vi "SP Convert 4.0 - 4.1 to 4.2.vi"(0 "S Parameter 4.0 - 4.1 Test Parameters":T3={"Tag"="", "Stimulus"={"Use Instrument Settings"=FALSE, "Sweep Type"=enum."Linear", "Sweep"=[{"Fstart, MHz"=500.0, "Fstop, MHz"=1500.0, "Points"=201}], "Blank Frequencies"=FALSE, "Power, dBm"=999.0, "IFBW, Hz"=-1.0, "Sweep Time, s"=-1.0}, "Measurements"=[{"Channel"=0, "Parameters"=[]}], "Datasheets"={"Datasheets to Generate"=[], "Print Datasheets"=FALSE}, "Quick Mode"=FALSE, "Display"={"Retain Settings"=FALSE, "Lock Control"=FALSE, "Plot Orientation"=enum."Single", "CH Controls"=[{"Trace Orientation"=enum."Overlay", "Frequency"={"Start"=500.0, "Stop"=1500.0, "Units"="MHz"}, "CH1Control"={"ChOn"=TRUE, "Measure"=0, "Format"=0, "Autoscale"=TRUE, "Reference"=0.0, "\nRefUnit"="dB/Div", "Position"=5.0, "Scale"=10.0, "ScaleUnit"="dB/Div", "LimitOn"=TRUE, "LimitFill"=FALSE, "Display Data"=0, "Show Markers"=FALSE, "SXX"=""}, "CH2Control"={"ChOn"=TRUE, "Measure"=0, "Format"=0, "Autoscale"=TRUE, "Reference"=0.0, "\nRefUnit"="dB/Div", "Position"=5.0, "Scale"=10.0, "ScaleUnit"="dB/Div", "LimitOn"=TRUE, "LimitFill"=FALSE, "Display Data"=0, "Show Markers"=FALSE, "SXX"=""}, "Markers"=[]}, {"Trace Orientation"=enum."Overlay", "Frequency"={"Start"=500.0, "Stop"=1500.0, "Units"="MHz"}, "CH1Control"={"ChOn"=TRUE, "Measure"=0, "Format"=0, "Autoscale"=TRUE, "Reference"=0.0, "\nRefUnit"="dB/Div", "Position"=5.0, "Scale"=10.0, "ScaleUnit"="dB/Div", "LimitOn"=TRUE, "LimitFill"=FALSE, "Display Data"=0, "Show Markers"=FALSE, "SXX"=""}, "CH2Control"={"ChOn"=TRUE, "Measure"=0, "Format"=0, "Autoscale"=TRUE, "Reference"=0.0, "\nRefUnit"="dB/Div", "Position"=5.0, "Scale"=10.0, "ScaleUnit"="dB/Div", "LimitOn"=TRUE, "LimitFill"=FALSE, "Display Data"=0, "Show Markers"=FALSE, "SXX"=""}, "Markers"=[]}, {"Trace Orientation"=enum."Overlay", "Frequency"={"Start"=500.0, "Stop"=1500.0, "Units"="MHz"}, "CH1Control"={"ChOn"=TRUE, "Measure"=0, "Format"=0, "Autoscale"=TRUE, "Reference"=0.0, "\nRefUnit"="dB/Div", "Position"=5.0, "Scale"=10.0, "ScaleUnit"="dB/Div", "LimitOn"=TRUE, "LimitFill"=FALSE, "Display Data"=0, "Show Markers"=FALSE, "SXX"=""}, "CH2Control"={"ChOn"=TRUE, "Measure"=0, "Format"=0, "Autoscale"=TRUE, "Reference"=0.0, "\nRefUnit"="dB/Div", "Position"=5.0, "Scale"=10.0, "ScaleUnit"="dB/Div", "LimitOn"=TRUE, "LimitFill"=FALSE, "Display Data"=0, "Show Markers"=FALSE, "SXX"=""}, "Markers"=[]}, {"Trace Orientation"=enum."Overlay", "Frequency"={"Start"=500.0, "Stop"=1500.0, "Units"="MHz"}, "CH1Control"={"ChOn"=TRUE, "Measure"=0, "Format"=0, "Autoscale"=TRUE, "Reference"=0.0, "\nRefUnit"="dB/Div", "Position"=5.0, "Scale"=10.0, "ScaleUnit"="dB/Div", "LimitOn"=TRUE, "LimitFill"=FALSE, "Display Data"=0, "Show Markers"=FALSE, "SXX"=""}, "CH2Control"={"ChOn"=TRUE, "Measure"=0, "Format"=0, "Autoscale"=TRUE, "Reference"=0.0, "\nRefUnit"="dB/Div", "Position"=5.0, "Scale"=10.0, "ScaleUnit"="dB/Div", "LimitOn"=TRUE, "LimitFill"=FALSE, "Display Data"=0, "Show Markers"=FALSE, "SXX"=""}, "Markers"=[]}], "Formatted Data"=FALSE}, "Auto Select"=TRUE, "Calibration"={"State"=FALSE, "String"=""}} {"Stimulus"."Sweep Time, s" format="%.3g"; "Display"."CH Controls"."Frequency"."Stop" format="%.3g"; "Display"."CH Controls"."Frequency"."Start" format="%.3g"; "Display"."CH Controls"."CH2Control"."Reference" format="%#.2g"; "Display"."CH Controls"."CH2Control"."Display Data" items=["Data", "Memory", "Data/Memory"]; "Display"."CH Controls"."CH2Control"."Format" items=["Log Mag", "Phase", "Delay", "Smith", "Polar", "Lin Mag", "SWR", "Loss", "Real", "Imaginary"]; "Display"."CH Controls"."CH2Control"."Scale" min=0.001 step=1.0 format="%#.2g"; "Display"."CH Controls"."CH2Control"."Position" min=0.0 max=10.0; "Display"."CH Controls"."CH1Control"."Reference" format="%#.2g"; "Display"."CH Controls"."CH1Control"."Display Data" items=["Data", "Memory", "Data/Memory"]; "Display"."CH Controls"."CH1Control"."Format" items=["Log Mag", "Phase", "Delay", "Smith", "Polar", "Lin Mag", "SWR", "Loss", "Real", "Imaginary"]; "Display"."CH Controls"."CH1Control"."Scale" min=0.001 step=1.0 format="%#.2g"; "Display"."CH Controls"."CH1Control"."Position" min=0.0 max=10.0; "Measurements"."Parameters"."Limits"."Run" min=1 step=1; "Measurements"."Channel" min=0 max=32 step=1}) -> (1 "QuickMode":i8, 2 "S Parameter 4.2 Test Parameters":T2={"Stimulus"={"Use Instrument Settings"=FALSE, "Blank Frequencies"=FALSE, "Sweep Type"=enum."Linear", "Sweep"={"Fstart"=0.0, "Fstop"=0.0, "Units"=enum."Hz", "Points"=2}, "Power (dBm)"=999.0, "IFBW (Hz)"=-1.0, "Sweep Time (s)"=-1.0}, "Measurement"={"Auto Select"=TRUE, "Data Source"=enum."VNA", "Ports"=2, "Calibration"={"State"=FALSE, "String"=""}, "Parameters"=[]}, "De-Embed"={"De-Embed"=FALSE, "Adapters"=[]}, "Display"={"Lock Control"=FALSE, "Retain Settings"=TRUE, "Formatted Data"=FALSE, "Plot Orientation"=enum."Single", "Plot Controls"=[{"Trace Orientation"=enum."Overlay", "Frequency"={"Change Frequency"=FALSE, "Start"=500.0, "Stop"=1500.0, "Units"=enum."MHz"}, "Markers (MHz)"=[], "Traces"=[{"Trace On"=TRUE, "Measure"=0, "Format"=0, "Autoscale"=TRUE, "Reference"=0.0, "\nRefUnit"="dB/Div", "Position"=5.0, "Scale"=10.0, "ScaleUnit"="dB/Div", "LimitOn"=TRUE, "LimitFill"=FALSE, "Display Data"=0, "Show Markers"=FALSE, "SXX"=""}, {"Trace On"=TRUE, "Measure"=0, "Format"=0, "Autoscale"=TRUE, "Reference"=0.0, "\nRefUnit"="dB/Div", "Position"=5.0, "Scale"=10.0, "ScaleUnit"="dB/Div", "LimitOn"=TRUE, "LimitFill"=FALSE, "Display Data"=0, "Show Markers"=FALSE, "SXX"=""}]}, {"Trace Orientation"=enum."Overlay", "Frequency"={"Change Frequency"=FALSE, "Start"=500.0, "Stop"=1500.0, "Units"=enum."MHz"}, "Markers (MHz)"=[], "Traces"=[{"Trace On"=TRUE, "Measure"=0, "Format"=0, "Autoscale"=TRUE, "Reference"=0.0, "\nRefUnit"="dB/Div", "Position"=5.0, "Scale"=10.0, "ScaleUnit"="dB/Div", "LimitOn"=TRUE, "LimitFill"=FALSE, "Display Data"=0, "Show Markers"=FALSE, "SXX"=""}, {"Trace On"=TRUE, "Measure"=0, "Format"=0, "Autoscale"=TRUE, "Reference"=0.0, "\nRefUnit"="dB/Div", "Position"=5.0, "Scale"=10.0, "ScaleUnit"="dB/Div", "LimitOn"=TRUE, "LimitFill"=FALSE, "Display Data"=0, "Show Markers"=FALSE, "SXX"=""}]}, {"Trace Orientation"=enum."Overlay", "Frequency"={"Change Frequency"=FALSE, "Start"=500.0, "Stop"=1500.0, "Units"=enum."MHz"}, "Markers (MHz)"=[], "Traces"=[{"Trace On"=TRUE, "Measure"=0, "Format"=0, "Autoscale"=TRUE, "Reference"=0.0, "\nRefUnit"="dB/Div", "Position"=5.0, "Scale"=10.0, "ScaleUnit"="dB/Div", "LimitOn"=TRUE, "LimitFill"=FALSE, "Display Data"=0, "Show Markers"=FALSE, "SXX"=""}, {"Trace On"=TRUE, "Measure"=0, "Format"=0, "Autoscale"=TRUE, "Reference"=0.0, "\nRefUnit"="dB/Div", "Position"=5.0, "Scale"=10.0, "ScaleUnit"="dB/Div", "LimitOn"=TRUE, "LimitFill"=FALSE, "Display Data"=0, "Show Markers"=FALSE, "SXX"=""}]}, {"Trace Orientation"=enum."Overlay", "Frequency"={"Change Frequency"=FALSE, "Start"=500.0, "Stop"=1500.0, "Units"=enum."MHz"}, "Markers (MHz)"=[], "Traces"=[{"Trace On"=TRUE, "Measure"=0, "Format"=0, "Autoscale"=TRUE, "Reference"=0.0, "\nRefUnit"="dB/Div", "Position"=5.0, "Scale"=10.0, "ScaleUnit"="dB/Div", "LimitOn"=TRUE, "LimitFill"=FALSE, "Display Data"=0, "Show Markers"=FALSE, "SXX"=""}, {"Trace On"=TRUE, "Measure"=0, "Format"=0, "Autoscale"=TRUE, "Reference"=0.0, "\nRefUnit"="dB/Div", "Position"=5.0, "Scale"=10.0, "ScaleUnit"="dB/Div", "LimitOn"=TRUE, "LimitFill"=FALSE, "Display Data"=0, "Show Markers"=FALSE, "SXX"=""}]}]}, "Limits"=[], "Datasheets"=[]} {"Measurement"."Parameters"."Channel" min=0 max=32 step=1; "Stimulus"."Sweep Time (s)" format="%.3g"; "Display"."Plot Controls"."Traces"."Reference" format="%#.2g"; "Display"."Plot Controls"."Traces"."Display Data" items=["Data", "Memory", "Data/Memory"]; "Display"."Plot Controls"."Traces"."Format" items=["Log Mag", "Phase", "Delay", "Smith", "Polar", "Lin Mag", "SWR", "Loss", "Real", "Imaginary"]; "Display"."Plot Controls"."Traces"."Scale" min=0.001 step=1.0 format="%#.2g"; "Display"."Plot Controls"."Traces"."Position" min=0.0 max=10.0; "Display"."Plot Controls"."Frequency"."Stop" format="%.3g"; "Display"."Plot Controls"."Frequency"."Start" format="%.3g"})   [LabVIEW 2011]
uses:
  TypeDefs/SP Test Parameters v3.2 and 4.0-4.1.ctl
  TypeDefs/SP Test Parameters v4.2.ctl
  TypeDefs/SP Format.ctl
panel:
  in  "Format":T1
  # "Div"
  # "Div"
  # "Div"
  # "="
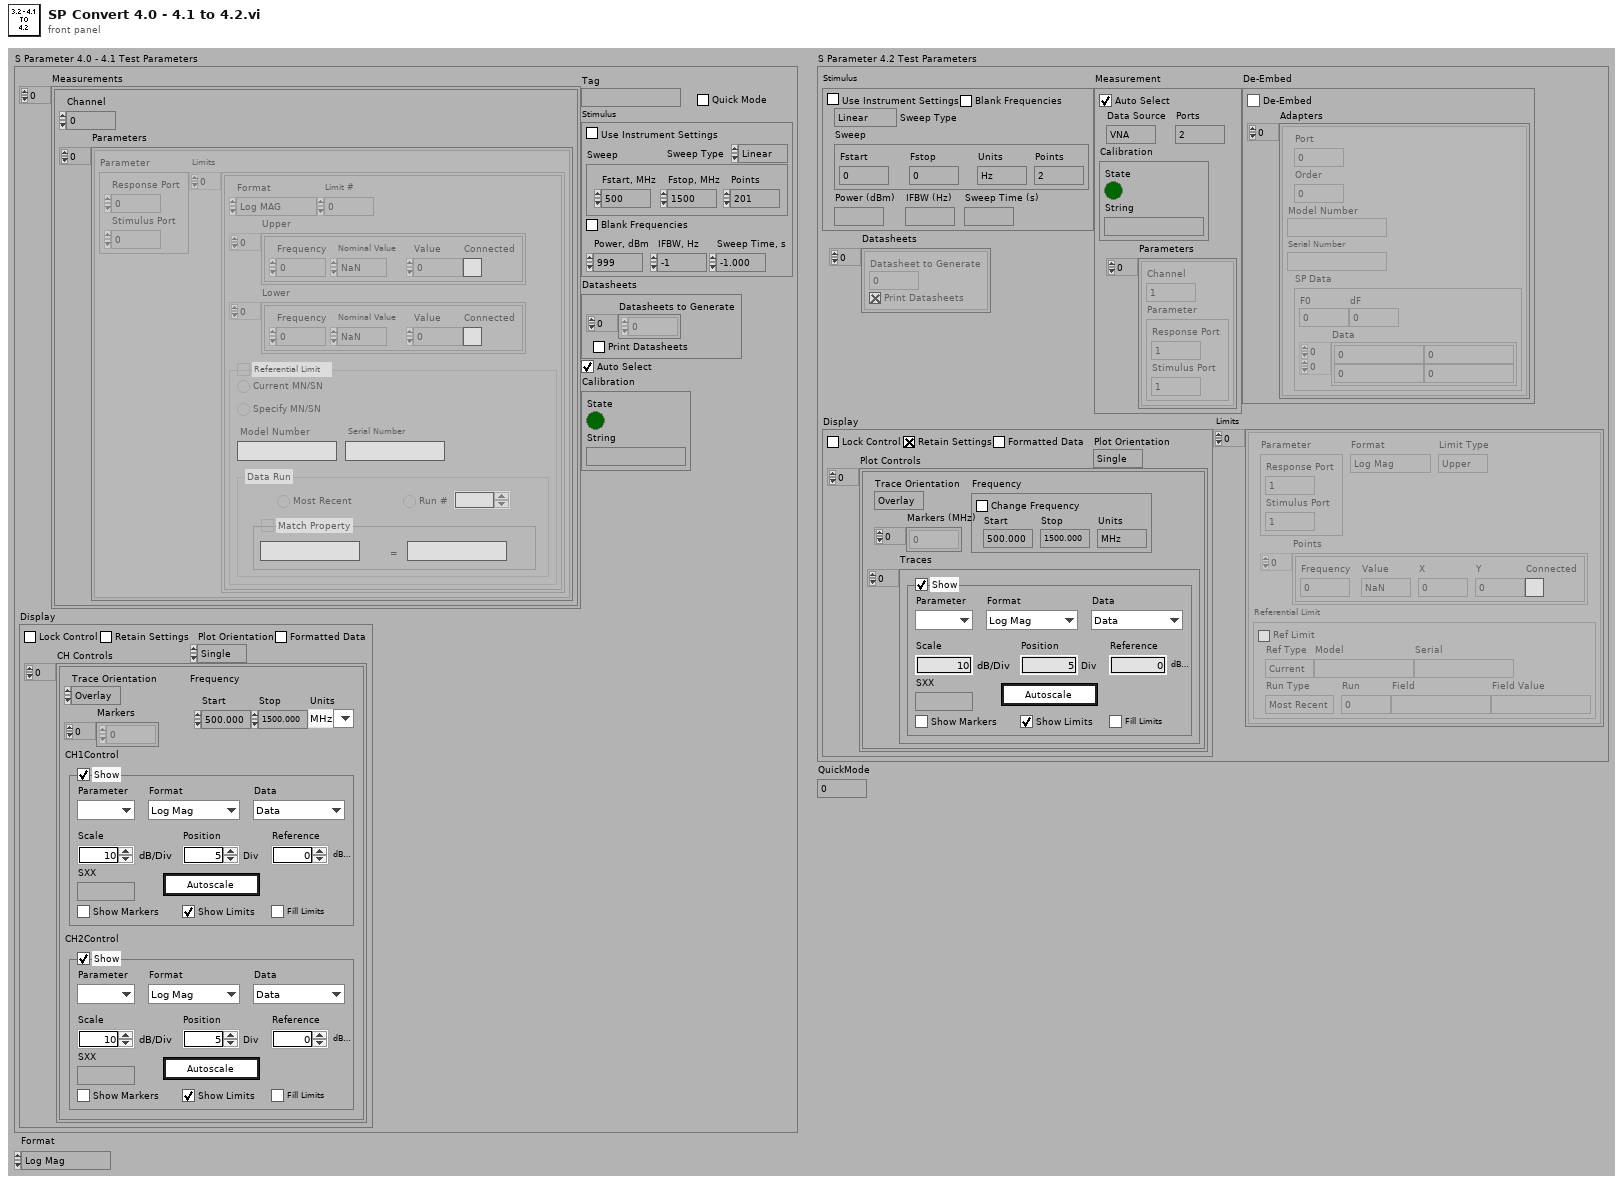
[diagram p1: front panel]
types:
  T1 = typedef "SP Format.ctl" = enum16{"Log Mag", "Lin Mag", "SWR", "Phase", "Expanded Phase", "Delay", "Insertion Loss", "Isolation", "Return Loss"}
  T2 = typedef "SP Test Parameters v4.2.ctl" = cluster{"Stimulus":cluster{"Use Instrument Settings":bool, "Blank Frequencies":bool, "Sweep Type":enum32{"Linear", "Logarithmic", "List", "Power", "CW"}, "Sweep":cluster{"Fstart":dbl, "Fstop":dbl, "Units":enum16{"Hz", "kHz", "MHz", "GHz"}, "Points":i32}, "Power (dBm)":dbl, "IFBW (Hz)":dbl, "Sweep Time (s)":dbl}, "Measurement":cluster{"Auto Select":bool, "Data Source":enum16{"VNA", "Data File"}, "Ports":i8, "Calibration":cluster{"State":bool, "String":string}, "Parameters":cluster{"Channel":i8, "Parameter":cluster{"Stimulus Port":i8, "Response Port":i8}}[]}, "De-Embed":cluster{"De-Embed":bool, "Adapters":cluster{"Port":i8, "Order":i8, "Model Number":string, "Serial Number":string, "SP Data":cluster{"F0":dbl, "dF":dbl, "Data":cdb[][]}}[]}, "Display":cluster{"Lock Control":bool, "Retain Settings":bool, "Formatted Data":bool, "Plot Orientation":enum32{"Single", "Dual", "Quad"}, "Plot Controls":cluster{"Trace Orientation":enum32{"Overlay", "Split"}, "Frequency":cluster{"Change Frequency":bool, "Start":dbl, "Stop":dbl, "Units":enum16{"Hz", "kHz", "MHz", "GHz"}}, "Markers (MHz)":dbl[], "Traces":cluster{"Trace On":bool, "Measure":i32, "Format":i32, "Autoscale":bool, "Reference":dbl, "\nRefUnit":string, "Position":dbl, "Scale":dbl, "ScaleUnit":string, "LimitOn":bool, "LimitFill":bool, "Display Data":u16, "Show Markers":bool, "SXX":string}[]}[]}, "Limits":cluster{"Parameter":cluster{"Stimulus Port":i8, "Response Port":i8}, "Format":enum16{"Log Mag", "Lin Mag", "SWR", "Phase", "Delay", "Insertion Loss", "Isolation", "Return Loss"}, "Limit Type":enum16{"Upper", "Lower", "Delta"}, "Points":cluster{"Frequency":dbl, "Value":dbl, "X":dbl, "Y":dbl, "Connected":bool}[], "Referential Limit":cluster{"Ref Limit":bool, "Ref Type":enum16{"Current", "Specify"}, "Model":string, "Serial":string, "Run Type":enum16{"Most Recent", "Run #", "Match Field"}, "Run":i32, "Field":string, "Field Value":string}}[], "Datasheets":cluster{"Datasheet to Generate":i32, "Print Datasheets":bool}[]}
  T3 = typedef "SP Test Parameters v3.2 and 4.0-4.1.ctl" = cluster{"Tag":string, "Stimulus":cluster{"Use Instrument Settings":bool, "Sweep Type":enum32{"Linear", "Log", "List", "Power", "CW"}, "Sweep":cluster{"Fstart, MHz":dbl, "Fstop, MHz":dbl, "Points":i32}[], "Blank Frequencies":bool, "Power, dBm":dbl, "IFBW, Hz":dbl, "Sweep Time, s":dbl}, "Measurements":cluster{"Channel":i8, "Parameters":cluster{"Parameter":cluster{"Stimulus Port":i8, "Response Port":i8}, "Limits":cluster{"Format":enum16{"Log MAG", "Lin MAG", "VSWR", "Phase", "Delay", "Insertion Loss", "Isolation", "Return Loss"}, "Upper":cluster{"Frequency":dbl, "Nominal Value":dbl, "Value":dbl, "Connected":bool}[], "Lower":cluster{"Frequency":dbl, "Nominal Value":dbl, "Value":dbl, "Connected":bool}[], "Limit #":i32, "Ref Limit":bool, "Ref Type":enum32{"Current", "Specify"}, "Model":string, "Serial":string, "Run Type":enum32{"Most Recent", "Run #"}, "Run":i32, "Match Property":bool, "Property":string, "Property Value":string}[]}[]}[], "Datasheets":cluster{"Datasheets to Generate":i32[], "Print Datasheets":bool}, "Quick Mode":bool, "Display":cluster{"Retain Settings":bool, "Lock Control":bool, "Plot Orientation":enum32{"Single", "Dual", "Quad"}, "CH Controls":cluster{"Trace Orientation":enum32{"Overlay", "Split"}, "Frequency":cluster{"Start":dbl, "Stop":dbl, "Units":string}, "CH1Control":cluster{"ChOn":bool, "Measure":i32, "Format":i32, "Autoscale":bool, "Reference":dbl, "\nRefUnit":string, "Position":dbl, "Scale":dbl, "ScaleUnit":string, "LimitOn":bool, "LimitFill":bool, "Display Data":u16, "Show Markers":bool, "SXX":string}, "CH2Control":cluster{"ChOn":bool, "Measure":i32, "Format":i32, "Autoscale":bool, "Reference":dbl, "\nRefUnit":string, "Position":dbl, "Scale":dbl, "ScaleUnit":string, "LimitOn":bool, "LimitFill":bool, "Display Data":u16, "Show Markers":bool, "SXX":string}, "Markers":dbl[]}[], "Formatted Data":bool}, "Auto Select":bool, "Calibration":cluster{"State":bool, "String":string}}
  T4 = enum32{"Linear", "Logarithmic", "List", "Power", "CW"}
  T5 = cluster{"Datasheet to Generate":i32, "Print Datasheets":bool}[]
  T6 = cluster{"Trace Orientation":enum32{"Overlay", "Split"}, "Frequency":cluster{"Change Frequency":bool, "Start":dbl, "Stop":dbl, "Units":enum16{"Hz", "kHz", "MHz", "GHz"}}, "Markers (MHz)":dbl[], "Traces":cluster{"Trace On":bool, "Measure":i32, "Format":i32, "Autoscale":bool, "Reference":dbl, "\nRefUnit":string, "Position":dbl, "Scale":dbl, "ScaleUnit":string, "LimitOn":bool, "LimitFill":bool, "Display Data":u16, "Show Markers":bool, "SXX":string}[]}[]
  T7 = cluster{"Channel":i8, "Parameter":cluster{"Stimulus Port":i8, "Response Port":i8}}[]
  T8 = cluster{"Parameter":cluster{"Stimulus Port":i8, "Response Port":i8}, "Format":enum16{"Log Mag", "Lin Mag", "SWR", "Phase", "Delay", "Insertion Loss", "Isolation", "Return Loss"}, "Limit Type":enum16{"Upper", "Lower", "Delta"}, "Points":cluster{"Frequency":dbl, "Value":dbl, "X":dbl, "Y":dbl, "Connected":bool}[], "Referential Limit":cluster{"Ref Limit":bool, "Ref Type":enum16{"Current", "Specify"}, "Model":string, "Serial":string, "Run Type":enum16{"Most Recent", "Run #", "Match Field"}, "Run":i32, "Field":string, "Field Value":string}}[]
  T9 = cluster{"Parameter":cluster{"Stimulus Port":i8, "Response Port":i8}, "Format":enum16{"Log Mag", "Lin Mag", "SWR", "Phase", "Delay", "Insertion Loss", "Isolation", "Return Loss"}, "Limit Type":enum16{"Upper", "Lower", "Delta"}, "Points":cluster{"Frequency":dbl, "Value":dbl, "X":dbl, "Y":dbl, "Connected":bool}[], "Referential Limit":cluster{"Ref Limit":bool, "Ref Type":enum16{"Current", "Specify"}, "Model":string, "Serial":string, "Run Type":enum16{"Most Recent", "Run #", "Match Field"}, "Run":i32, "Field":string, "Field Value":string}}
  T10 = cluster{"Frequency":dbl, "Value":dbl, "X":dbl, "Y":dbl, "Connected":bool}[]
  T11 = cluster{"Trace Orientation":enum32{"Overlay", "Split"}, "Frequency":cluster{"Change Frequency":bool, "Start":dbl, "Stop":dbl, "Units":enum16{"Hz", "kHz", "MHz", "GHz"}}, "Markers (MHz)":dbl[], "Traces":cluster{"Trace On":bool, "Measure":i32, "Format":i32, "Autoscale":bool, "Reference":dbl, "\nRefUnit":string, "Position":dbl, "Scale":dbl, "ScaleUnit":string, "LimitOn":bool, "LimitFill":bool, "Display Data":u16, "Show Markers":bool, "SXX":string}[]}
  T12 = cluster{"Fstart, MHz":dbl, "Fstop, MHz":dbl, "Points":i32}[]
  T13 = cluster{"Datasheets to Generate":i32[], "Print Datasheets":bool}
  T14 = cluster{"Trace Orientation":enum32{"Overlay", "Split"}, "Frequency":cluster{"Start":dbl, "Stop":dbl, "Units":string}, "CH1Control":cluster{"ChOn":bool, "Measure":i32, "Format":i32, "Autoscale":bool, "Reference":dbl, "\nRefUnit":string, "Position":dbl, "Scale":dbl, "ScaleUnit":string, "LimitOn":bool, "LimitFill":bool, "Display Data":u16, "Show Markers":bool, "SXX":string}, "CH2Control":cluster{"ChOn":bool, "Measure":i32, "Format":i32, "Autoscale":bool, "Reference":dbl, "\nRefUnit":string, "Position":dbl, "Scale":dbl, "ScaleUnit":string, "LimitOn":bool, "LimitFill":bool, "Display Data":u16, "Show Markers":bool, "SXX":string}, "Markers":dbl[]}[]
  T15 = cluster{"Channel":i8, "Parameters":cluster{"Parameter":cluster{"Stimulus Port":i8, "Response Port":i8}, "Limits":cluster{"Format":enum16{"Log MAG", "Lin MAG", "VSWR", "Phase", "Delay", "Insertion Loss", "Isolation", "Return Loss"}, "Upper":cluster{"Frequency":dbl, "Nominal Value":dbl, "Value":dbl, "Connected":bool}[], "Lower":cluster{"Frequency":dbl, "Nominal Value":dbl, "Value":dbl, "Connected":bool}[], "Limit #":i32, "Ref Limit":bool, "Ref Type":enum32{"Current", "Specify"}, "Model":string, "Serial":string, "Run Type":enum32{"Most Recent", "Run #"}, "Run":i32, "Match Property":bool, "Property":string, "Property Value":string}[]}[]}[]
  T16 = cluster{"Trace On":bool, "Measure":i32, "Format":i32, "Autoscale":bool, "Reference":dbl, "\nRefUnit":string, "Position":dbl, "Scale":dbl, "ScaleUnit":string, "LimitOn":bool, "LimitFill":bool, "Display Data":u16, "Show Markers":bool, "SXX":string}[]
  T17 = cluster{"Frequency":dbl, "Value":dbl, "X":dbl, "Y":dbl, "Connected":bool}
  T18 = cluster{"Channel":i8, "Parameter":cluster{"Stimulus Port":i8, "Response Port":i8}}
  T19 = enum16{"Log Mag", "Lin Mag", "SWR", "Phase", "Delay", "Insertion Loss", "Isolation", "Return Loss"}
  T20 = cluster{"Parameter":cluster{"Stimulus Port":i8, "Response Port":i8}, "Limits":cluster{"Format":enum16{"Log MAG", "Lin MAG", "VSWR", "Phase", "Delay", "Insertion Loss", "Isolation", "Return Loss"}, "Upper":cluster{"Frequency":dbl, "Nominal Value":dbl, "Value":dbl, "Connected":bool}[], "Lower":cluster{"Frequency":dbl, "Nominal Value":dbl, "Value":dbl, "Connected":bool}[], "Limit #":i32, "Ref Limit":bool, "Ref Type":enum32{"Current", "Specify"}, "Model":string, "Serial":string, "Run Type":enum32{"Most Recent", "Run #"}, "Run":i32, "Match Property":bool, "Property":string, "Property Value":string}[]}[]
  T21 = cluster{"Format":enum16{"Log MAG", "Lin MAG", "VSWR", "Phase", "Delay", "Insertion Loss", "Isolation", "Return Loss"}, "Upper":cluster{"Frequency":dbl, "Nominal Value":dbl, "Value":dbl, "Connected":bool}[], "Lower":cluster{"Frequency":dbl, "Nominal Value":dbl, "Value":dbl, "Connected":bool}[], "Limit #":i32, "Ref Limit":bool, "Ref Type":enum32{"Current", "Specify"}, "Model":string, "Serial":string, "Run Type":enum32{"Most Recent", "Run #"}, "Run":i32, "Match Property":bool, "Property":string, "Property Value":string}[]
  T22 = enum16{"Log MAG", "Lin MAG", "VSWR", "Phase", "Delay", "Insertion Loss", "Isolation", "Return Loss"}
  T23 = cluster{"Frequency":dbl, "Nominal Value":dbl, "Value":dbl, "Connected":bool}[]
  T24 = cluster{"Frequency":dbl, "Nominal Value":dbl, "Value":dbl, "Connected":bool}
  T25 = cluster{"Trace On":bool, "Measure":i32, "Format":i32, "Autoscale":bool, "Reference":dbl, "\nRefUnit":string, "Position":dbl, "Scale":dbl, "ScaleUnit":string, "LimitOn":bool, "LimitFill":bool, "Display Data":u16, "Show Markers":bool, "SXX":string}
  T26 = cluster{"Fstart, MHz":dbl, "Fstop, MHz":dbl, "Points":i32}
  T27 = typedef "SP Display Data.ctl" = u16
  T28 = cluster{"Datasheet to Generate":i32, "Print Datasheets":bool}
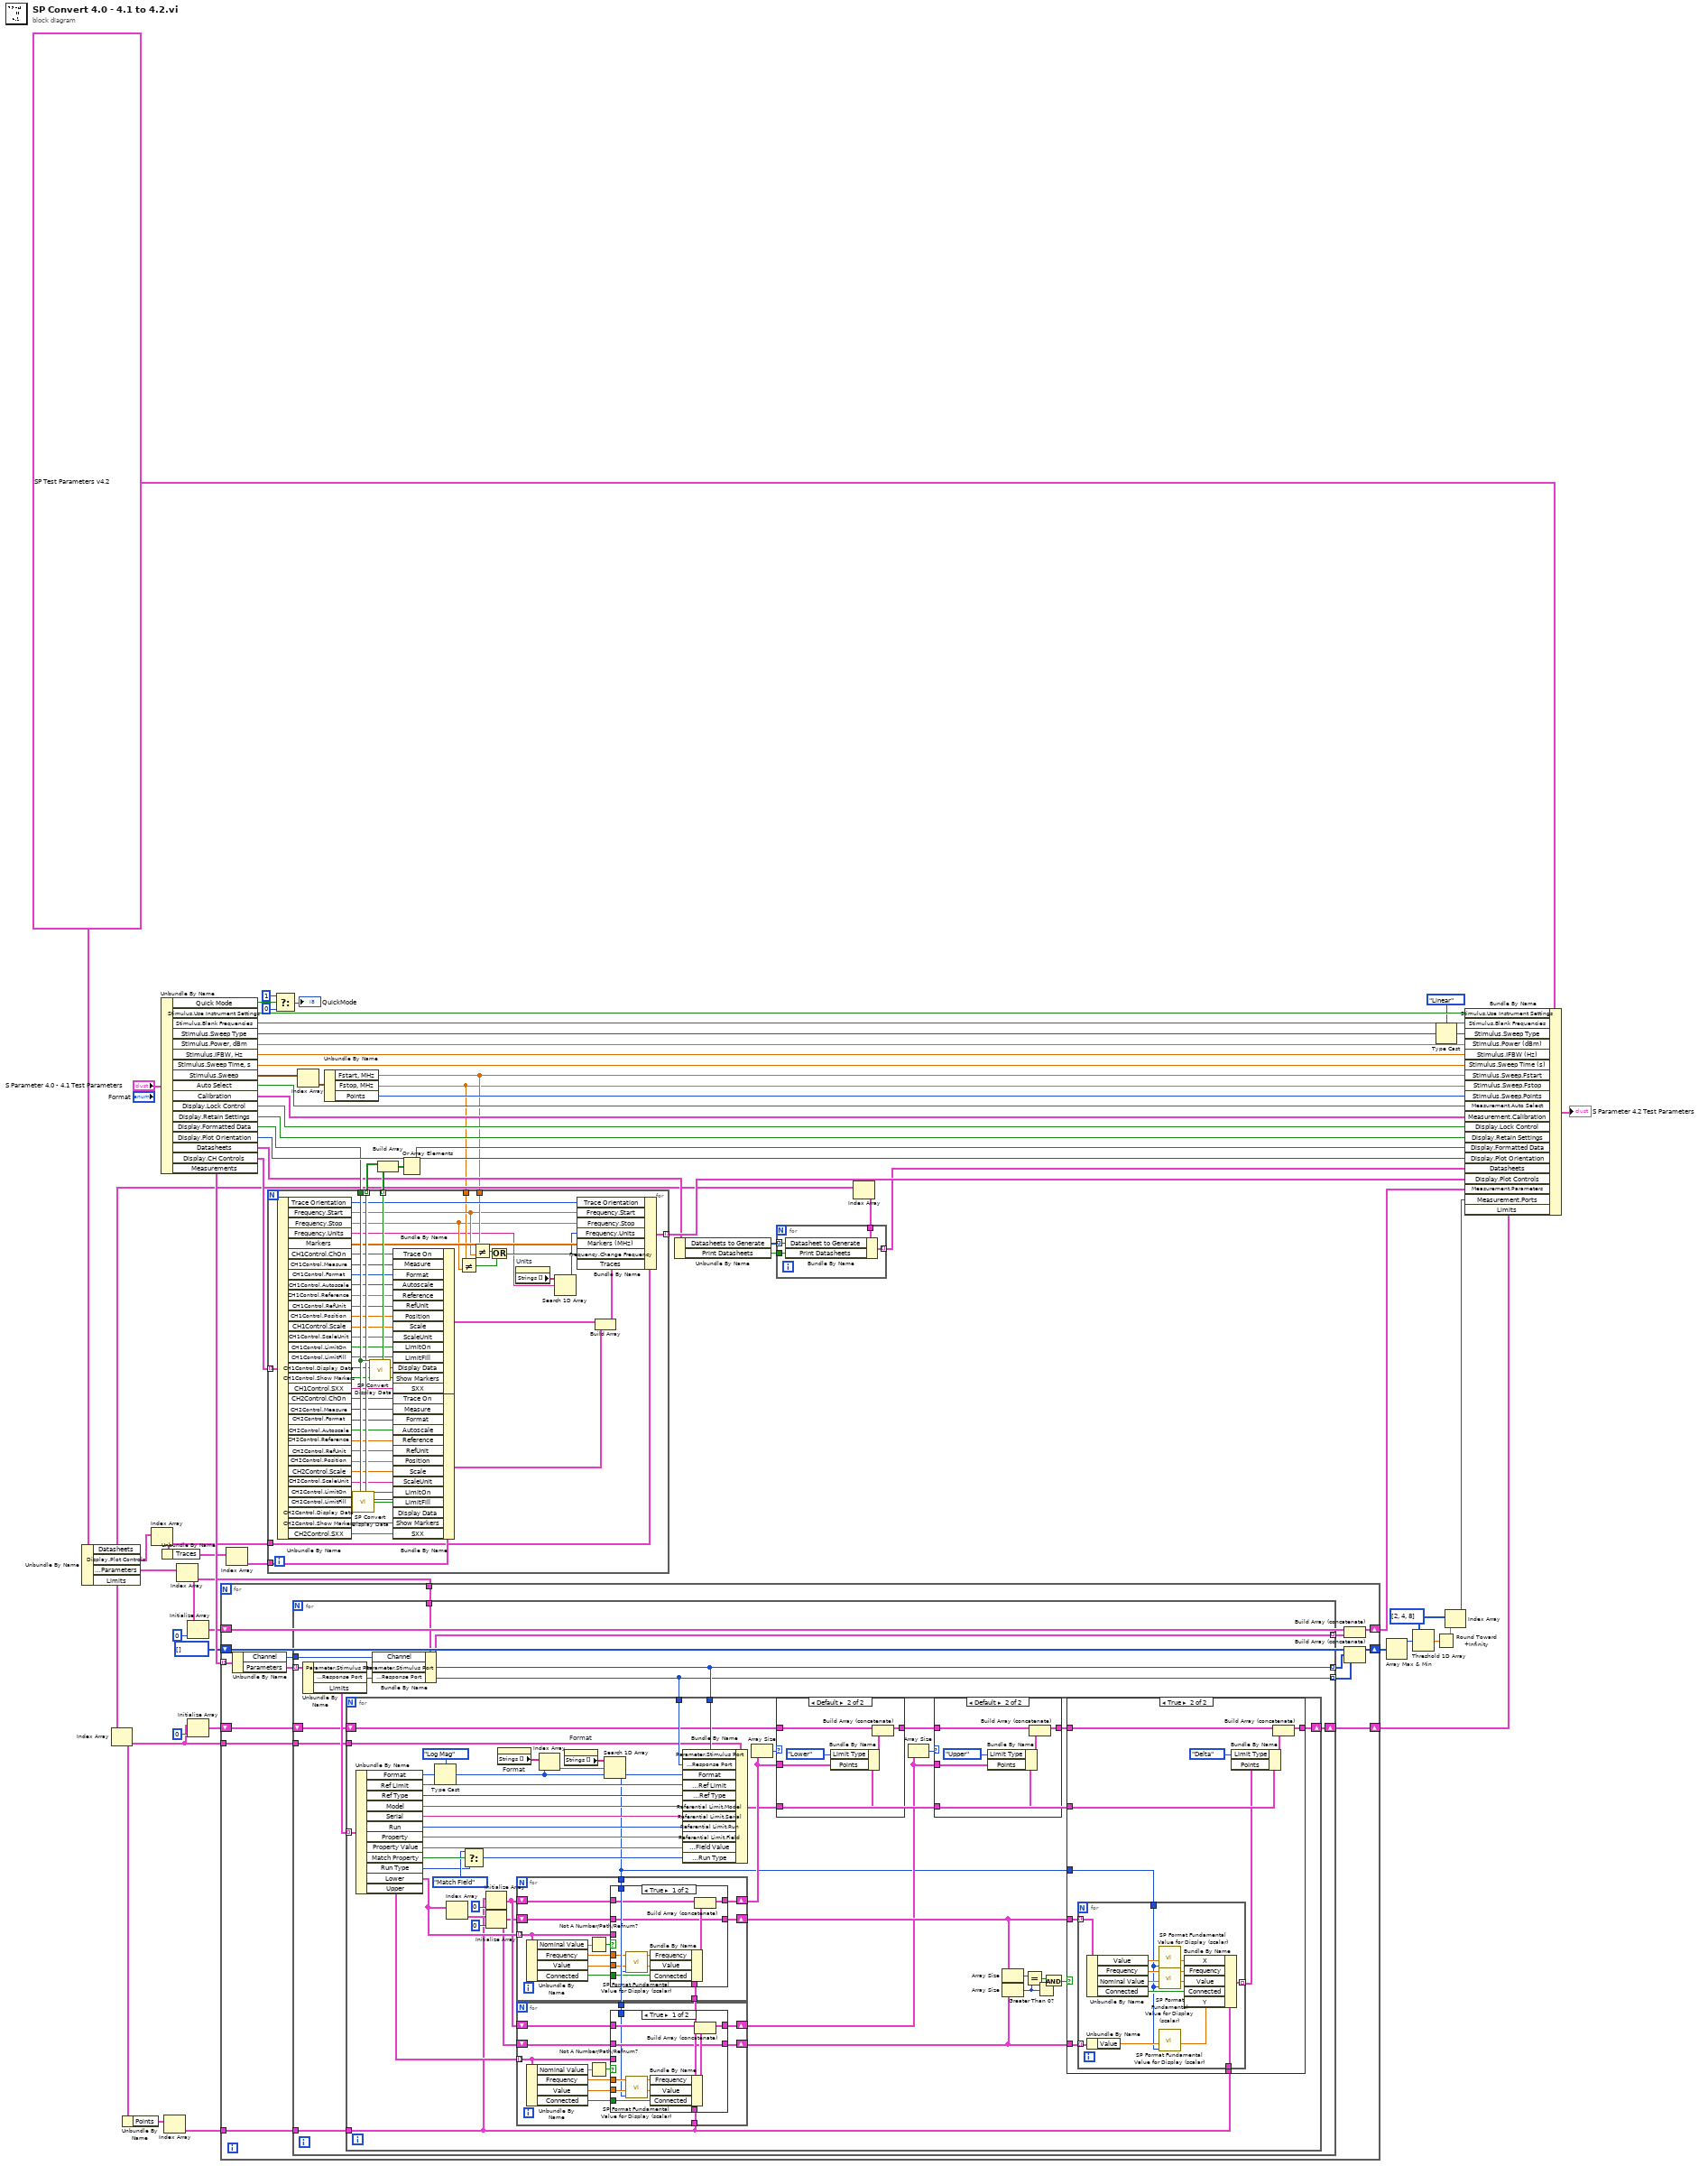
[diagram p0: block diagram]
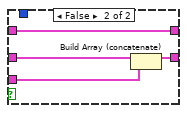
[diagram p2: hidden frame]
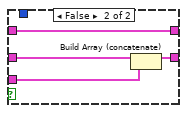
[diagram p6: hidden frame]
diagram:
  w30 = i8[] [2, 4, 8]
  w42 = T2 {"Stimulus"={"Use Instrument Settings"=FALSE, "Blank Frequencies"=FALSE, "Sweep Type"=enum."Linear", "Sweep"={"Fstart"=0.0, "Fstop"=0.0, "Units"=enum."Hz", "Points"=2}, "Power (dBm)"=999.0, "IFBW (Hz)"=-1.0, "Sweep Time (s)"=-1.0}, "Measurement"={"Auto Select"=TRUE, "Data Source"=enum."VNA", "Ports"=2, "Calibration"={"State"=FALSE, "String"=""}, "Parameters"=[]}, "De-Embed"={"De-Embed"=FALSE, "Adapters"=[]}, "Display"={"Lock Control"=FALSE, "Retain Settings"=TRUE, "Formatted Data"=FALSE, "Plot Orientation"=enum."Single", "Plot Controls"=[{"Trace Orientation"=enum."Overlay", "Frequency"={"Change Frequency"=FALSE, "Start"=500.0, "Stop"=1500.0, "Units"=enum."MHz"}, "Markers (MHz)"=[], "Traces"=[{"Trace On"=TRUE, "Measure"=0, "Format"=0, "Autoscale"=TRUE, "Reference"=0.0, "\nRefUnit"="dB/Div", "Position"=5.0, "Scale"=10.0, "ScaleUnit"="dB/Div", "LimitOn"=TRUE, "LimitFill"=FALSE, "Display Data"=0, "Show Markers"=FALSE, "SXX"=""}, {"Trace On"=TRUE, "Measure"=0, "Format"=0, "Autoscale"=TRUE, "Reference"=0.0, "\nRefUnit"="dB/Div", "Position"=5.0, "Scale"=10.0, "ScaleUnit"="dB/Div", "LimitOn"=TRUE, "LimitFill"=FALSE, "Display Data"=0, "Show Markers"=FALSE, "SXX"=""}]}, {"Trace Orientation"=enum."Overlay", "Frequency"={"Change Frequency"=FALSE, "Start"=500.0, "Stop"=1500.0, "Units"=enum."MHz"}, "Markers (MHz)"=[], "Traces"=[{"Trace On"=TRUE, "Measure"=0, "Format"=0, "Autoscale"=TRUE, "Reference"=0.0, "\nRefUnit"="dB/Div", "Position"=5.0, "Scale"=10.0, "ScaleUnit"="dB/Div", "LimitOn"=TRUE, "LimitFill"=FALSE, "Display Data"=0, "Show Markers"=FALSE, "SXX"=""}, {"Trace On"=TRUE, "Measure"=0, "Format"=0, "Autoscale"=TRUE, "Reference"=0.0, "\nRefUnit"="dB/Div", "Position"=5.0, "Scale"=10.0, "ScaleUnit"="dB/Div", "LimitOn"=TRUE, "LimitFill"=FALSE, "Display Data"=0, "Show Markers"=FALSE, "SXX"=""}]}, {"Trace Orientation"=enum."Overlay", "Frequency"={"Change Frequency"=FALSE, "Start"=500.0, "Stop"=1500.0, "Units"=enum."MHz"}, "Markers (MHz)"=[], "Traces"=[{"Trace On"=TRUE, "Measure"=0, "Format"=0, "Autoscale"=TRUE, "Reference"=0.0, "\nRefUnit"="dB/Div", "Position"=5.0, "Scale"=10.0, "ScaleUnit"="dB/Div", "LimitOn"=TRUE, "LimitFill"=FALSE, "Display Data"=0, "Show Markers"=FALSE, "SXX"=""}, {"Trace On"=TRUE, "Measure"=0, "Format"=0, "Autoscale"=TRUE, "Reference"=0.0, "\nRefUnit"="dB/Div", "Position"=5.0, "Scale"=10.0, "ScaleUnit"="dB/Div", "LimitOn"=TRUE, "LimitFill"=FALSE, "Display Data"=0, "Show Markers"=FALSE, "SXX"=""}]}, {"Trace Orientation"=enum."Overlay", "Frequency"={"Change Frequency"=FALSE, "Start"=500.0, "Stop"=1500.0, "Units"=enum."MHz"}, "Markers (MHz)"=[], "Traces"=[{"Trace On"=TRUE, "Measure"=0, "Format"=0, "Autoscale"=TRUE, "Reference"=0.0, "\nRefUnit"="dB/Div", "Position"=5.0, "Scale"=10.0, "ScaleUnit"="dB/Div", "LimitOn"=TRUE, "LimitFill"=FALSE, "Display Data"=0, "Show Markers"=FALSE, "SXX"=""}, {"Trace On"=TRUE, "Measure"=0, "Format"=0, "Autoscale"=TRUE, "Reference"=0.0, "\nRefUnit"="dB/Div", "Position"=5.0, "Scale"=10.0, "ScaleUnit"="dB/Div", "LimitOn"=TRUE, "LimitFill"=FALSE, "Display Data"=0, "Show Markers"=FALSE, "SXX"=""}]}]}, "Limits"=[], "Datasheets"=[]} ("S Parameter Test Parameters")
  n1 = Unbundle By Name(w42) -> ("Datasheets"=w13:T5, "Display.Plot Controls"=w18:T6, "Measurement.Parameters"=w39:T7, "Limits"=w26:T8)
  n2 = Index Array(array=w26) -> (element=w23:T9)  [unwired: 1 in]
  n3 = Unbundle By Name(w23) -> ("Points"=w27:T10)
  n4 = Index Array(array=w18) -> (element=w17:T11)  [unwired: 1 in]
  n5 = Unbundle By Name("S Parameter 4.0 - 4.1 Test Parameters") -> ("Quick Mode"=w9:bool, "Stimulus.Use Instrument Settings"=w57:bool, "Stimulus.Blank Frequencies"=w56:bool, "Stimulus.Sweep Type"=w1:enum32{"Linear", "Log", "List", "Power", "CW"}, "Stimulus.Power, dBm"=w55:dbl, "Stimulus.IFBW, Hz"=w54:dbl, "Stimulus.Sweep Time, s"=w53:dbl, "Stimulus.Sweep"=w52:T12, "Auto Select"=w49:bool, "Calibration"=w48:cluster{"State":bool, "String":string}, "Display.Lock Control"=w47:bool, "Display.Retain Settings"=w46:bool, "Display.Formatted Data"=w44:bool, "Display.Plot Orientation"=w45:enum32{"Single", "Dual", "Quad"}, "Datasheets"=w15:T13, "Display.CH Controls"=w41:T14, "Measurements"=w40:T15)
  n6 = Unbundle By Name(w17) -> ("Traces"=w19:T16)
  n7 = Index Array(array=w27) -> (element=w25:T17)  [unwired: 1 in]
  n8 = Index Array(array=w39) -> (element=w38:T18)  [unwired: 1 in]
  n9 = Initialize Array(w38, 0 ("dimension size")) -> (w36:T7)
  n10 = Initialize Array(w23, 0 ("dimension size")) -> (w22:T8)
  n11 = for {
    tunnel: w40 -> [w77] mode=indexing
    tunnel: w38 -> [w76]
    shift-right: [w71] -> w33
    shift-left: w36 -> [w72]
    shift-right: [w68] -> w34
    shift-left: i8[] [] -> [w69]
    tunnel: w25 -> [w66]
    tunnel: w23 -> [w65]
    shift-right: [w63] -> w21
    shift-left: w22 -> [w64]
    n12 = Unbundle By Name(w77) -> ("Channel"=w75:i8, "Parameters"=w74:T20)
    n13 = for {
      tunnel: w76 -> [w88]
      tunnel: w75 -> [w87]
      tunnel: w74 -> [w86] mode=indexing
      tunnel: [w85] -> w73 mode=indexing
      tunnel: [w83] -> w67 mode=indexing
      tunnel: [w82] -> w70 mode=indexing
      tunnel: w66 -> [w81]
      tunnel: w65 -> [w80]
      shift-right: [w78] -> w63
      shift-left: w64 -> [w79]
      n14 = Unbundle By Name(w86) -> ("Parameter.Stimulus Port"=w83:i8, "Parameter.Response Port"=w82:i8, "Limits"=w84:T21)
      n15 = for {
        tunnel: w84 -> [w134] mode=indexing
        tunnel: w83 -> [w123]
        tunnel: w82 -> [w122]
        tunnel: w81 -> [w96]
        tunnel: w80 -> [w114]
        shift-right: [w103] -> w78
        shift-left: w79 -> [w113]
        n16 = Unbundle By Name(w134) -> ("Format"=w93:T22, "Ref Limit"=w124:bool, "Ref Type"=w102:enum32{"Current", "Specify"}, "Model"=w125:string, "Serial"=w126:string, "Run"=w127:i32, "Property"=w132:string, "Property Value"=w133:string, "Match Property"=w131:bool, "Run Type"=w129:enum32{"Most Recent", "Run #"}, "Lower"=w121:T23, "Upper"=w99:T23)
        n17 = Type Cast(type=T19."Log Mag" ("Format"), x=w93) -> (*(type *) &x=w89:T19)
        n18 = Index Array(array=w121) -> (element=w118:T24)  [unwired: 1 in]
        n19 = Select(t=enum32{"Most Recent", "Run #", "Match Field"}."Match Field" ("Run Type"), s=w131, f=w129) -> (s? t:f=w128:enum32{"Most Recent", "Run #", "Match Field"})
        n20 = Initialize Array(w96, 0 ("dimension size")) -> (w101:T10)
        n21 = Initialize Array(w118, 0 ("dimension size")) -> (w100:T23)
        n22 = property on="Format" class="Enum (strict)"() -> ("Strings []"=w94:string[])  [unwired: 2 in, 2 out]
        n23 = Index Array(array=w94, index=w89) -> (element=w91:string)
        n24 = property on="Format" class="Enum (strict)"() -> ("Strings []"=w92:string[])  [unwired: 2 in, 2 out]
        n25 = Search 1D Array(1D array=w92, element=w91) -> (index of element=w90:i32)  [unwired: 1 out]
        n26 = for {
          tunnel: w121 -> [w202] mode=indexing
          shift-right: [w204] -> w111
          shift-left: w101 -> [w205]
          shift-right: [w201] -> w115
          shift-left: w100 -> [w203]
          tunnel: w96 -> [w200]
          tunnel: w90 -> [w199]
          n27 = Unbundle By Name(w202) -> ("Nominal Value"=w207:dbl, "Frequency"=w209:dbl, "Value"=w208:dbl, "Connected"=w210:bool)
          n28 = Not A Number/Path/Refnum?(number/path/refnum=w207) -> (NaN/Path/Refnum?=w206:bool)
          n29 = case shown="True" w206 {
            tunnel: w210 -> [w212 _]
            tunnel: w209 -> [w220 _]
            tunnel: w208 -> [w214 _]
            tunnel: w205 -> [w218 w224]
            tunnel: [w217 w224] -> w204
            tunnel: w203 -> [w216 w223]
            tunnel: w202 -> [_ w222]
            tunnel: [w216 w221] -> w201
            tunnel: w200 -> [w215 _]
            tunnel: w199 -> [w211 _]
            frame True {
              n30 = call "SP Format Fundamental Value for Display (scalar).vi"("Format"=w211, "Stored Value (0, linear)"=w214) -> ("Display Value"=w213:dbl)  [unwired: 5 out]
              n31 = Bundle By Name(cluster=w215, "Frequency"=w220, "Value"=w213, "Connected"=w212) -> (w219:T17)
              n32 = Build Array (concatenate)(w218, w219) -> (w217:T10)
            }
            frame False {
              n33 = Build Array (concatenate)(w223, w222) -> (w221:T23)
            }
          }
        }
        n34 = for {
          tunnel: w99 -> [w138] mode=indexing
          shift-right: [w140] -> w97
          shift-left: w101 -> [w141]
          shift-right: [w137] -> w98
          shift-left: w100 -> [w139]
          tunnel: w96 -> [w136]
          tunnel: w90 -> [w135]
          n35 = Unbundle By Name(w138) -> ("Nominal Value"=w143:dbl, "Frequency"=w145:dbl, "Value"=w144:dbl, "Connected"=w146:bool)
          n36 = Not A Number/Path/Refnum?(number/path/refnum=w143) -> (NaN/Path/Refnum?=w142:bool)
          n37 = case shown="True" w142 {
            tunnel: w146 -> [w148 _]
            tunnel: w145 -> [w156 _]
            tunnel: w144 -> [w150 _]
            tunnel: w141 -> [w154 w160]
            tunnel: [w153 w160] -> w140
            tunnel: w139 -> [w152 w159]
            tunnel: w138 -> [_ w158]
            tunnel: [w152 w157] -> w137
            tunnel: w136 -> [w151 _]
            tunnel: w135 -> [w147 _]
            frame True {
              n38 = call "SP Format Fundamental Value for Display (scalar).vi"("Format"=w147, "Stored Value (0, linear)"=w150) -> ("Display Value"=w149:dbl)  [unwired: 5 out]
              n39 = Bundle By Name(cluster=w151, "Frequency"=w156, "Value"=w149, "Connected"=w148) -> (w155:T17)
              n40 = Build Array (concatenate)(w154, w155) -> (w153:T10)
            }
            frame False {
              n41 = Build Array (concatenate)(w159, w158) -> (w157:T23)
            }
          }
        }
        n42 = Bundle By Name(cluster=w114, "Parameter.Stimulus Port"=w123, "Parameter.Response Port"=w122, "Format"=w89, "Referential Limit.Ref Limit"=w124, "Referential Limit.Ref Type"=w102, "Referential Limit.Model"=w125, "Referential Limit.Serial"=w126, "Referential Limit.Run"=w127, "Referential Limit.Field"=w132, "Referential Limit.Field Value"=w133, "Referential Limit.Run Type"=w128) -> (w104:T9)
        n43 = Array Size(array=w111) -> (size(s)=w112:i32)
        n44 = case shown="Default" w112 {
          tunnel: w113 -> [w168 w174]
          tunnel: w104 -> [_ w173]
          tunnel: w111 -> [_ w172]
          tunnel: [w168 w169] -> w109
          frame 0 {
          }
          frame Default {
            n45 = Bundle By Name(cluster=w173, "Limit Type"=enum16{"Upper", "Lower", "Delta"}."Lower", "Points"=w172) -> (w171:T9)
            n46 = Build Array (concatenate)(w174, w171) -> (w169:T8)
          }
        }
        n47 = Array Size(array=w97) -> (size(s)=w110:i32)
        n48 = case shown="Default" w110 {
          tunnel: w109 -> [w161 w167]
          tunnel: w104 -> [_ w166]
          tunnel: w97 -> [_ w165]
          tunnel: [w161 w162] -> w105
          frame 0 {
          }
          frame Default {
            n49 = Bundle By Name(cluster=w166, "Limit Type"=enum16{"Upper", "Lower", "Delta"}."Upper", "Points"=w165) -> (w164:T9)
            n50 = Build Array (concatenate)(w167, w164) -> (w162:T8)
          }
        }
        n51 = Array Size(array=w115) -> (size(s)=w108:i32)
        n52 = Array Size(array=w98) -> (size(s)=w107:i32)
        n53 = Equal?(x=w108, y=w107) -> (x = y?=w106:bool)
        n54 = Greater Than 0?(x=w107) -> (x > 0?=w117:bool)
        n55 = And(x=w106, y=w117) -> (x .and. y?=w116:bool)
        n56 = case shown="True" w116 {
          tunnel: w115 -> [_ w185]
          tunnel: w98 -> [_ w184]
          tunnel: w105 -> [w175 w181]
          tunnel: w104 -> [_ w180]
          tunnel: [w175 w178] -> w103
          tunnel: w96 -> [_ w177]
          tunnel: w90 -> [_ w176]
          frame False {
          }
          frame True {
            n57 = for {
              tunnel: w185 -> [w198] mode=indexing
              tunnel: w184 -> [w195] mode=indexing
              tunnel: [w194] -> w179 mode=indexing
              tunnel: w177 -> [w193]
              tunnel: w176 -> [w186]
              n58 = Unbundle By Name(w198) -> ("Value"=w192:dbl, "Frequency"=w196:dbl, "Nominal Value"=w191:dbl, "Connected"=w197:bool)
              n59 = Unbundle By Name(w195) -> ("Value"=w190:dbl)
              n60 = call "SP Format Fundamental Value for Display (scalar).vi"("Format"=w186, "Stored Value (0, linear)"=w192) -> ("Display Value"=w187:dbl)  [unwired: 5 out]
              n61 = call "SP Format Fundamental Value for Display (scalar).vi"("Format"=w186, "Stored Value (0, linear)"=w191) -> ("Display Value"=w188:dbl)  [unwired: 5 out]
              n62 = call "SP Format Fundamental Value for Display (scalar).vi"("Format"=w186, "Stored Value (0, linear)"=w190) -> ("Display Value"=w189:dbl)  [unwired: 5 out]
              n63 = Bundle By Name(cluster=w193, "X"=w187, "Frequency"=w196, "Value"=w188, "Connected"=w197, "Y"=w189) -> (w194:T17)
            }
            n64 = Bundle By Name(cluster=w180, "Limit Type"=enum16{"Upper", "Lower", "Delta"}."Delta", "Points"=w179) -> (w182:T9)
            n65 = Build Array (concatenate)(w181, w182) -> (w178:T8)
          }
        }
      }
      n66 = Bundle By Name(cluster=w88, "Channel"=w87, "Parameter.Stimulus Port"=w83, "Parameter.Response Port"=w82) -> (w85:T18)
    }
    n67 = Build Array (concatenate)(w72, w73) -> (w71:T7)
    n68 = Build Array (concatenate)(w69, w67, w70) -> (w68:i8[])
  }
  n69 = Index Array(array=w19) -> (element=w20:T25)  [unwired: 1 in]
  n70 = Select(t=i8 1 ("QuickMode"), s=w9, f=i8 0 ("QuickMode")) -> (s? t:f=→"QuickMode":i8)
  n71 = Index Array(array=w52) -> (element=w51:T26)  [unwired: 1 in]
  n72 = Unbundle By Name(w51) -> ("Fstart, MHz"=w5:dbl, "Fstop, MHz"=w4:dbl, "Points"=w50:i32)
  n73 = for {
    tunnel: w41 -> [w273] mode=indexing
    tunnel: w44 -> [w276]
    tunnel: [w275] -> w59 mode=indexing
    tunnel: [w274] -> w60 mode=indexing
    tunnel: w20 -> [w272]
    tunnel: w17 -> [w239]
    tunnel: [w236] -> w16 mode=indexing
    tunnel: w5 -> [w231]
    tunnel: w4 -> [w229]
    n74 = Unbundle By Name(w273) -> ("Trace Orientation"=w235:enum32{"Overlay", "Split"}, "Frequency.Start"=w230:dbl, "Frequency.Stop"=w228:dbl, "Frequency.Units"=w226:string, "Markers"=w237:dbl[], "CH1Control.ChOn"=w271:bool, "CH1Control.Measure"=w270:i32, "CH1Control.Format"=w269:i32, "CH1Control.Autoscale"=w267:bool, "CH1Control.Reference"=w268:dbl, "CH1Control.RefUnit"=w266:string, "CH1Control.Position"=w265:dbl, "CH1Control.Scale"=w264:dbl, "CH1Control.ScaleUnit"=w263:string, "CH1Control.LimitOn"=w262:bool, "CH1Control.LimitFill"=w261:bool, "CH1Control.Display Data"=w242:u16, "CH1Control.Show Markers"=w260:bool, "CH1Control.SXX"=w259:string, "CH2Control.ChOn"=w258:bool, "CH2Control.Measure"=w257:i32, "CH2Control.Format"=w256:i32, "CH2Control.Autoscale"=w255:bool, "CH2Control.Reference"=w254:dbl, "CH2Control.RefUnit"=w252:string, "CH2Control.Position"=w253:dbl, "CH2Control.Scale"=w251:dbl, "CH2Control.ScaleUnit"=w250:string, "CH2Control.LimitOn"=w249:bool, "CH2Control.LimitFill"=w248:bool, "CH2Control.Display Data"=w245:u16, "CH2Control.Show Markers"=w247:bool, "CH2Control.SXX"=w246:string)
    n75 = call "SP Convert Display Data.vi"("Old Formatted Data"=w276, "Old Data Display"=w245) -> ("New Data Display"=w244:T27, "New Formatted Data"=w274:bool)  [unwired: 8 out]
    n76 = call "SP Convert Display Data.vi"("Old Formatted Data"=w276, "Old Data Display"=w242) -> ("New Data Display"=w243:T27, "New Formatted Data"=w275:bool)  [unwired: 8 out]
    n77 = Bundle By Name(cluster=w272, "Trace On"=w271, "Measure"=w270, "Format"=w269, "Autoscale"=w267, "Reference"=w268, "RefUnit"=w266, "Position"=w265, "Scale"=w264, "ScaleUnit"=w263, "LimitOn"=w262, "LimitFill"=w261, "Display Data"=w243, "Show Markers"=w260, "SXX"=w259) -> (w241:T25)
    n78 = Bundle By Name(cluster=w272, "Trace On"=w258, "Measure"=w257, "Format"=w256, "Autoscale"=w255, "Reference"=w254, "RefUnit"=w252, "Position"=w253, "Scale"=w251, "ScaleUnit"=w250, "LimitOn"=w249, "LimitFill"=w248, "Display Data"=w244, "Show Markers"=w247, "SXX"=w246) -> (w240:T25)
    n79 = Not Equal?(x=w229, y=w228) -> (x != y?=w233:bool)
    n80 = Not Equal?(x=w231, y=w230) -> (x != y?=w234:bool)
    n81 = Or(x=w234, y=w233) -> (x .or. y?=w232:bool)
    n82 = property on="Units" class="Enum (strict)"() -> ("Strings []"=w227:string[])  [unwired: 2 in, 2 out]
    n83 = Search 1D Array(1D array=w227, element=w226) -> (index of element=w225:i32)  [unwired: 1 out]
    n84 = Build Array(w241, w240) -> (w238:T16)
    n85 = Bundle By Name(cluster=w239, "Trace Orientation"=w235, "Frequency.Start"=w230, "Frequency.Stop"=w228, "Frequency.Units"=w225, "Markers (MHz)"=w237, "Frequency.Change Frequency"=w232, "Traces"=w238) -> (w236:T11)
  }
  n86 = Build Array(w60, w59) -> (w58:bool[][])
  n87 = Or Array Elements(Boolean array=w58) -> (logical OR=w43:bool)
  n88 = Unbundle By Name(w15) -> ("Datasheets to Generate"=w14:i32[], "Print Datasheets"=w11:bool)
  n89 = Index Array(array=w13) -> (element=w12:T28)  [unwired: 1 in]
  n90 = for {
    tunnel: w14 -> [w279] mode=indexing
    tunnel: w12 -> [w280]
    tunnel: w11 -> [w278]
    tunnel: [w277] -> w10 mode=indexing
    n91 = Bundle By Name(cluster=w280, "Datasheet to Generate"=w279, "Print Datasheets"=w278) -> (w277:T28)
  }
  n92 = Array Max & Min(array=w34) -> (max value=w29:i8)  [unwired: 3 out]
  n93 = Threshold 1D Array(2:w29, 3:w30) -> (0:w32:dbl)  [unwired: 1 out]
  n94 = Type Cast(type=T4."Linear" ("Stimulus.Sweep Type"), x=w1) -> (*(type *) &x=w3:T4)
  n95 = Round Toward +Infinity(x=w32) -> (ceil(x): smallest int >= x=w31:dbl)
  n96 = Index Array(array=w30, index=w31) -> (element=w28:i8)
  n97 = Bundle By Name(cluster=w42, "Stimulus.Use Instrument Settings"=w57, "Stimulus.Blank Frequencies"=w56, "Stimulus.Sweep Type"=w3, "Stimulus.Power (dBm)"=w55, "Stimulus.IFBW (Hz)"=w54, "Stimulus.Sweep Time (s)"=w53, "Stimulus.Sweep.Fstart"=w5, "Stimulus.Sweep.Fstop"=w4, "Stimulus.Sweep.Points"=w50, "Measurement.Auto Select"=w49, "Measurement.Calibration"=w48, "Display.Lock Control"=w47, "Display.Retain Settings"=w46, "Display.Formatted Data"=w43, "Display.Plot Orientation"=w45, "Datasheets"=w10, "Display.Plot Controls"=w16, "Measurement.Parameters"=w33, "Measurement.Ports"=w28, "Limits"=w21) -> (→"S Parameter 4.2 Test Parameters":T2)
